vi "HCalSet.vi"(1 "RH?":bool, 2 "Calibration In":u8[][](array[numeric])) -> (0 "Same Array Out":u8[][](array[numeric]))   [LabVIEW 2009]
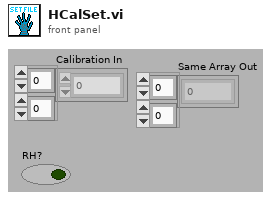
[diagram p1: front panel]
types:
  T1 = enum16{"open", "replace", "create", "open or create", "replace or create", "replace or create with confirmation"}
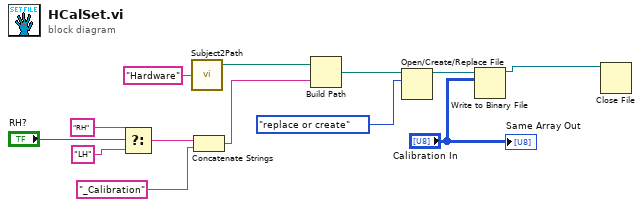
[diagram p0: block diagram]
diagram:
  n1 = Select(t="RH" ("name or relative path"), s="RH?", f="LH" ("name or relative path")) -> (s? t:f=w5:string)
  n2 = call "Subject2Path.vi"("Subject Initials"="Hardware") -> ("Subject Root"=w12:path)  [unwired: 1 in, 2 out]
  n3 = Concatenate Strings(w5, "_Calibration" ("name or relative path")) -> (w3:string)
  n4 = Build Path(base path=w12, name or relative path=w3) -> (appended path=w11:path)
  n5 = Open/Create/Replace File(file path (use dialog)=w11, operation (0:open)=T1."replace or create") -> (refnum out=w9:refnum<file>)  [unwired: 4 in, 2 out]
  n6 = Write to Binary File(file (use dialog)=w9, data="Calibration In") -> (refnum out=w2:refnum<file>)  [unwired: 4 in, 2 out]
  n7 = Close File(refnum=w2) -> ()  [unwired: 1 in, 2 out]
  "Same Array Out" <- "Calibration In"
